vi "Set Slew Rates.vi"(0 "reference in":refnum<class "Simulated-PowerModule.lvclass">, 5 "Slew Rates":T1, 11 "Error In":errorcluster) -> (4 "reference out":refnum<class "Simulated-PowerModule.lvclass">, 15 "Error Out":errorcluster)   [LabVIEW 2023, in "Simulated-PowerModule.lvlib" / "Simulated-PowerModule.lvclass"]
uses:
  Simulated-PowerModule.lvclass
  builds/PowerModuleInterface/PowerModuleInterface.lvlibp/Classes/PowerModule_interface/Slew Rates.ctl
  builds/PowerModuleInterface/PowerModuleInterface.lvlibp/Classes/PowerModule_interface/PowerModuleInterface.lvclass
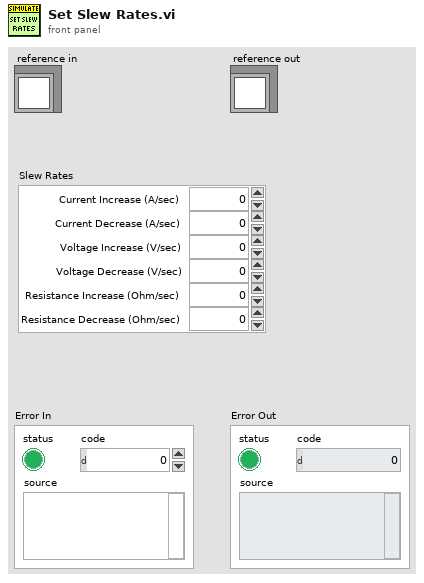
[diagram p1: front panel]
types:
  T1 = typedef "PowerModuleInterface.lvlibp/PowerModuleInterface.lvclass/Slew Rates.ctl" = cluster{"Current Decrease (A/sec)":dbl, "Current Increase (A/sec)":dbl, "Voltage Decrease (V/sec)":dbl, "Voltage Increase (V/sec)":dbl, "Resistance Decrease (Ohm/sec)":dbl, "Resistance Increase (Ohm/sec)":dbl}
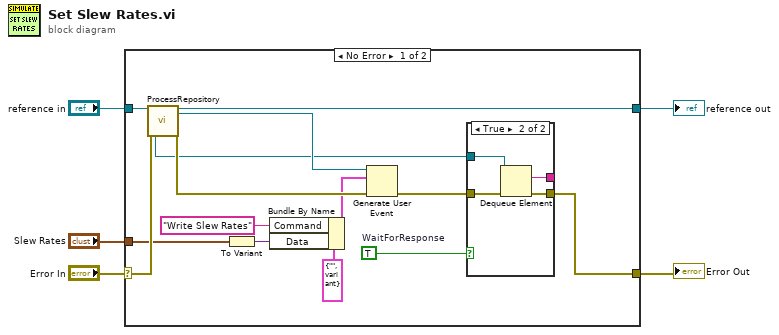
[diagram p0: block diagram]
diagram:
  n1 = case shown="No Error" "Error In" {
    selector: "Error In" -> [w19 w26]
    tunnel: [w12 w26] -> w4
    tunnel: [w17 w25] -> w2
    tunnel: "reference in" -> [w18 w25]
    tunnel: "Slew Rates" -> [w6 _]
    frame No Error {
      w15 = TRUE  # WaitForResponse
      n2 = call "ProcessRepository.vi"("reference in"=w18, "Error In"=w19) -> ("QueueFromProcess"=w9:refnum<queue>, "reference out"=w17:refnum<class "Simulated-PowerModule.lvclass">, "EventsToProcess"=w16:refnum<user-event>, "Error Out"=w13:errorcluster)  [unwired: 10 in, 4 out]
      n3 = To Variant(anything=w6) -> (Variant=w7:variant)
      n4 = Bundle By Name(cluster=cluster{"Command":string, "Data":variant} {"Command"="", "Data"=variant} ("MessageToProcess"), "Command"="Write Slew Rates", "Data"=w7) -> (w10:cluster{"Command":string, "Data":variant})
      n5 = Generate User Event(user event=w16, event data cluster=w10, error in=w13) -> (error out=w14:errorcluster)  [unwired: 1 in, 1 out]
      n6 = case shown="True" w15 {
        tunnel: w14 -> [w20 w24]
        tunnel: [_ w23] -> _
        tunnel: [w20 w22] -> w12
        tunnel: w9 -> [_ w21]
        frame False {
        }
        frame True {
          n7 = Dequeue Element(queue=w21, error in (no error)=w24) -> (element=w23:string, error out=w22:errorcluster)  [unwired: 1 in, 2 out]
        }
      }
    }
    frame Error {
    }
  }
  "Error Out" <- w4
  "reference out" <- w2
